vi "Implement IIR Cascade Filter (CDB).vi"(7 "Reset":bool, 8 "error in (no error)":errorcluster, 10 "IIR Filter Cluster":T1 {"Forward Coefficients" format="%0.4f"; "Reverse Coefficients" format="%0.4f"}, 11 "Waveform":waveform(cdb)) -> (0 "error out":errorcluster, 3 "Filtered Waveform":waveform(cdb))   [LabVIEW 2020, in "NI_MAPro.lvlib"]
uses:
  NI_MAPro.lvlib
  NI_MABase.lvlib
  NI_AALBase.lvlib
panel:
  in  "shift register type":cdb[](array[numeric]) format="%0.2f"
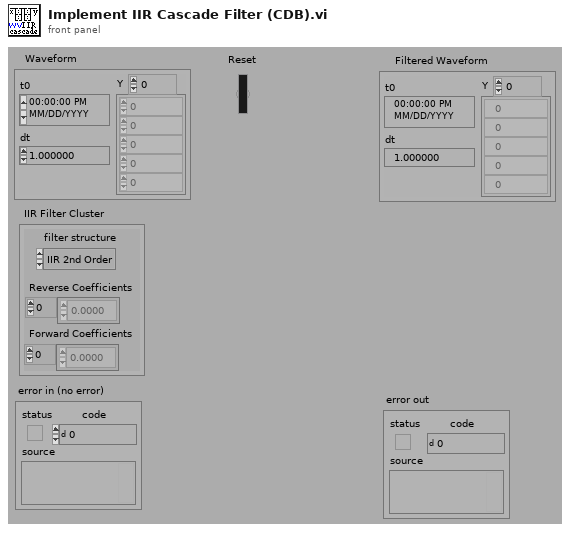
[diagram p1: front panel]
types:
  T1 = cluster{"filter structure":enum32{"IIR 2nd Order", "IIR 4th Order"}, "Reverse Coefficients":dbl[], "Forward Coefficients":dbl[]}
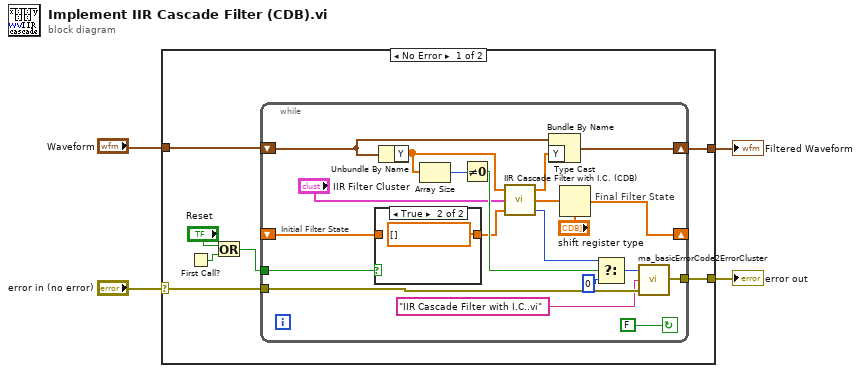
[diagram p0: block diagram]
diagram:
  n1 = case shown="No Error" "error in (no error)" {
    selector: "error in (no error)" -> [w10 w35]
    tunnel: [w11 w35] -> w3
    tunnel: [w9 w34] -> w2
    tunnel: "Waveform" -> [w8 w34]
    frame No Error {
      n2 = First Call?() -> (First Call?: T/F=w5:bool)
      n3 = Or(x="Reset", y=w5) -> (x .or. y?=w6:bool)
      n4 = while {
        tunnel: w10 -> [w19]
        tunnel: w6 -> [w21]
        tunnel: [w20] -> w11
        shift-left: w8 -> [w27]
        shift-right: [w28] -> w9
        shift-left: _ -> [w23]
        shift-right: [w30] -> _
        stop <- FALSE continue-if-true
        # "Final Filter State"
        # "Initial Filter State"
        n5 = case shown="True" w21 {
          tunnel: w23 -> [w32 _]
          tunnel: [w32 cdb[] [] ("shift register type")] -> w22
          frame False {
          }
          frame True {
          }
        }
        n6 = Unbundle By Name(w27) -> ("Y"=w14:cdb[])
        n7 = Array Size(array=w14) -> (size(s)=w13:i32)
        n8 = Not Equal To 0?(x=w13) -> (x != 0?=w31:bool)
        n9 = call "IIR Cascade Filter with I.C. (CDB).vi"("Initial Filter State"=w22, "IIR Filter Cluster"="IIR Filter Cluster", "X"=w14) -> ("error"=w15:i32, "Final Filter State"=w24:cdb[], "Filtered X"=w26:cdb[])
        n10 = Bundle By Name(cluster=w27, "Y"=w26) -> (w28:waveform(cdb))
        n11 = Type Cast(type="shift register type", x=w24) -> (*(type *) &x=w30:cdb[])
        n12 = Select(t=w15, s=w31, f=0) -> (s? t:f=w16:i32)
        n13 = call "ma_basicErrorCode2ErrorCluster.vi"("error in (no error)"=w19, "subVI name"="IIR Cascade Filter with I.C..vi", "Error Code"=w16) -> ("error out"=w20:errorcluster)
      }
    }
    frame Error {
    }
  }
  "error out" <- w3
  "Filtered Waveform" <- w2
